vi "HEWH Mass Removed.vi"(8 "Error In":errorcluster, 11 "UEF Calculated Values Output in":T1 {"Data Indexes"."15 sec after Draw Index" format="%#.2f"; "Data Indexes"."15 sec after Draw Timestamp" format="%#.2f"; "Data Indexes"."Test Start Timestamp" format="%.2f"; "Data Indexes"."Test End Timestamp" format="%.2f"; "Data Indexes"."T0 Timestamp" format="%.2f"; "Data Indexes"."Tsf Timestamp" format="%.2f"; "Data Indexes"."Tsu0 Timestamp" format="%.2f"; "Data Indexes"."Tmax1 Timestamp" format="%.2f"; "Data Indexes"."Draw Index Timestamp" format="%#.2f"; "Data Indexes"."Non-Draw Timestamp" format="%#.2f"; "Data Indexes"."Heating Timestamp" format="%#.2f"; "Data Indexes"."Start Energy (BTU-Gas)" format="%.6f"; "Data Indexes"."Start Watt Hours" format="%.6f"; "Static Data"."V - Volume of Wh (True)" format="%.5f"; "Static Data"."T-Ambinet Nominal (°F)" format="%.5f"; "Static Data"."T-Inlet Setpoint (°F)" format="%.5f"; "Static Data"."T-Wh Setpoint (°F)" format="%.5f"; "Sampled Data"."Qe (Wh)" format="%.5f"; "Sampled Data"."Tau stby2 (hr)" format="%.5f"; "Sampled Data"."Tastby2 (°F)" format="%.5f"; "Sampled Data"."Qf (BTU)" format="%.5f"; "Sampled Data"."Qe (BTU)" format="%.5f"; "Sampled Data"."Tmax1 (°F)" format="%.5f"; "Sampled Data"."T0 (°F)" format="%.5f"; "Sampled Data"."Qr (BTU)" format="%.5f"; "Sampled Data"."T 24(°F)" format="%.5f"; "Sampled Data"."T astby(°F)" format="%.5f"; "Sampled Data"."T tstby(°F)" format="%.5f"; "Sampled Data"."T su0(°F)" format="%.5f"; "Sampled Data"."T suf(°F)" format="%.5f"; "Sampled Data"."Tau stby_1 (hr)" format="%.5f"; "Sampled Data"."Qsuf (BTU)" format="%.5f"; "Sampled Data"."Qsu0 (BTU)" format="%.5f"; "Calculated Values"."Draw Bonus Volume (gal)" format="%.6f"; "Calculated Values"."Adjustment Factor" format="%.6f"; "Calculated Values"."T*avg_del(n-1)" format="%.6f"; "Calculated Values"."T*min(n-1)" format="%.6f"; "Calculated Values"."T*avg_del(n)" format="%.6f"; "Calculated Values"."Vn" format="%.6f"; "Calculated Values"."Qdm (BTU)" format="%.6f"; "Calculated Values"."QHWD (BTU)" format="%.6f"; "Calculated Values"."QHW (BTU)" format="%.6f"; "Calculated Values"."UEF" format="%.6f"; "Calculated Values"."QHW67 (BTU)" format="%.6f"; "Calculated Values"."Qda (BTU)" format="%.6f"; "Calculated Values"."Qd (BTU)" format="%.6f"; "Calculated Values"."Q (BTU)" format="%.6f"; "Calculated Values"."UA (BTU/(hr*F))" format="%.6f"; "Calculated Values"."Qhr (BTU/hr)" format="%.6f"; "Calculated Values"."Qstby (BTU)" format="%.6f"; "Calculated Values"."nu_r" format="%.6f"; "Calculated Values"."CpUEF (BTU/(lb*F))" format="%.6f"; "Calculated Values"."rho_nu (lb/gal)" format="%.6f"; "Calculated Values"."V1- Vol (Gal)" format="%.6f"; "Calculated Values"."M cluster mass removed (lb)" format="%.6f"; "Calculated Values"."Cp theoretical (BTU/(lbm °F))" format="%.6f"; "Calculated Values"."Tin1 - Mean Inlet 1st Cluster (°F)" format="%.6f"; "Calculated Values"."Tdel1-Mean Outlet 1st Cluster(°F)" format="%.6f"; "Calculated Values"."Cp 24 (BTU/(lb*F))" format="%.6f"; "Calculated Values"."Cp standby (BTU/(lb*F))" format="%.6f"; "Calculated Values"."Cp2 (BTU/(lb*F))" format="%.6f"; "Calculated Values"."Cp1 (BTU/(lb*F))" format="%.6f"; "Calculated Values"."rho 24 (lb/gal)" format="%.6f"; "Calculated Values"."rho standby (lb/gal)" format="%.6f"; "Calculated Values"."rho 2 (lb/gal)" format="%.6f"; "Calculated Values"."Density of cold water All (lbm/gal)" format="%#.3g"; "Calculated Values"."CpHW (BTU/(lbm °F))" format="%#.3g"; "Calculated Values"."Density of hot water All (lbm/gal)" format="%#.3g"; "Calculated Values"."Mass of water All (lbm)" format="%#.3f"}) -> (0 "Error Out":errorcluster, 3 "UEF Calculated Values Output out":T1={"Calculated Values"={"Draw Cluster - Actual (Gal)"=[], "Mass of water All (lbm)"=[], "Density of hot water All (lbm/gal)"=[], "CpHW (BTU/(lbm °F))"=[], "rho 2 (lb/gal)"=0.0, "rho standby (lb/gal)"=0.0, "rho 24 (lb/gal)"=0.0, "Cp1 (BTU/(lb*F))"=0.0, "Cp2 (BTU/(lb*F))"=0.0, "Cp standby (BTU/(lb*F))"=0.0, "Cp 24 (BTU/(lb*F))"=0.0, "nu_r"=0.0, "Qstby (BTU)"=0.0, "Qhr (BTU/hr)"=0.0, "UA (BTU/(hr*F))"=0.0, "Q (BTU)"=0.0, "Qd (BTU)"=0.0, "Qda (BTU)"=0.0, "QHW67 (BTU)"=0.0, "UEF"=0.0, "Tdel1-Mean Outlet 1st Cluster(°F)"=0.0, "Tin1 - Mean Inlet 1st Cluster (°F)"=0.0, "Cp theoretical (BTU/(lbm °F))"=0.0, "M cluster mass removed (lb)"=0.0, "V1- Vol (Gal)"=0.0, "Test Data -Start to End (Full Index)"=[], "rho_nu (lb/gal)"=0.0, "Density of cold water All (lbm/gal)"=[], "CpUEF (BTU/(lb*F))"=0.0, "QHW (BTU)"=0.0, "QHWD (BTU)"=0.0, "Qdm (BTU)"=0.0, "FHD-After 1 Hour (String)"=[], "Vn"=0.0, "T*avg_del(n)"=0.0, "Max Location"=0, "T*min(n-1)"=0.0, "T*avg_del(n-1)"=0.0, "Temp Greater than T*min(n-1)"=FALSE, "Adjustment Factor"=0.0, "Draw Bonus Volume (gal)"=0.0, "Flow Type - End Condition"=enum."ForcedDrawAfterHour"}, "Sampled Data"={"Cold Water Draw Amounts-(Gal)"=[], "T del_all - Outlet Temps (°F)"=[], "T in_all - Inlet Temps (°F)"=[], "Qsu0 (BTU)"=14385.3, "Qsuf (BTU)"=15959.6, "Tau stby_1 (hr)"=8.4, "T suf(°F)"=125.0, "T su0(°F)"=126.1, "T tstby(°F)"=124.2, "T astby(°F)"=68.8, "T 24(°F)"=123.2, "Qr (BTU)"=7657.9, "T0 (°F)"=124.7, "Tmax1 (°F)"=124.8, "Qe (BTU)"=32770.2, "Qf (BTU)"=0.0, "Tastby2 (°F)"=68.9, "RTD Out Full Data\nSet (Each Draw)"=[], "RTD IN Full Data\nSet (Each Draw)"=[], "Tau stby2 (hr)"=23.406, "Hot Water Draw Amounts-(Gal)"=[], "Cold Flow Rate (GPM)"=[], "Hot Flow Rate (GPM)"=[], "Softw Elapsed Time\n Full Data Set (Each Draw)"=[], "Cold Gal Total Full\nData Set (Each Draw)"=[], "Total Hot Draw Amount (Gal) "=0.0, "Total Cold Draw Amount (Gal)"=0.0, "Qe (Wh)"=0.0, "Hot Gal Total Full\nData Set (Each Draw)"=[]}, "Static Data"={"T-Wh Setpoint (°F)"=125.0, "T-Inlet Setpoint (°F)"=58.0, "T-Ambinet Nominal (°F)"=67.5, "V - Volume of Wh (True)"=46.0}, "Data Indexes"={"Test Start-Full Index (Found)"=0, "Header Length"=0, "Draw Index (Found)"=[], "Nr"=0, "Start Watt Hours"=0.0, "Tsu0 Index (Found)"=0, "Tsf Index (Found)"=0, "Start Energy (BTU-Gas)"=0.0, "Draws in Cluster"=0, "T0 Index-Full Index (Found)"=0, "Non-Draw Index (Found)"=[], "Tmax1 Index (Found)"=0, "Test End-Full Index (Found)"=0, "Heating Index (Found)"=[], "Heating Timestamp"=[], "Non-Draw Timestamp"=[], "Draw Index Timestamp"=[], "Tmax1 Timestamp"=0.0, "Tsu0 Timestamp"=0.0, "Tsf Timestamp"=0.0, "T0 Timestamp"=0.0, "Test End Timestamp"=0.0, "Test Start Timestamp"=0.0, "15 sec after Draw Timestamp"=[], "15 sec after Draw Index"=[], "Tmax1 Occurred During a Draw"=FALSE, "FHD Total Time (Sec)"=0.0, "Draw Pattern"=enum."Very Small Usage", "Standby Valid"=FALSE}, "Raw Data"={"Elapsed Time Index (DBL)"=0, "Software Elapsed Time Index (DBL)"=0, "TC Tree Avg Index (DBL)"=0, "Watt Hours -Wh Index (DBL)"=0, "Energy BTU Index (DBL)"=0, "Totalized Flow Index (DBL)"=0, "Flow Rate Index (DBL)"=0, "Program Status Index (Str)"=0, "RTDin Index (DBL)"=0, "RTDout Index (DBL)"=0, "RTDamb Index (DBL)"=0, "Test Data-Start to End DBL"=[], "Data Type"=enum."GEA Inlet Side Meter", "Heat Source Index (DBL)"=0, "Hot Water Rate GPM (DBL)"=0, "Hot Water Total - GAL (DBL)"=0, "FHD-After 1 hour"=[], "Humidity -% RH (DBL)"=0, "Voltage - V (DBL)"=0, "Draw Count (DBL)"=0, "Elapsed Time Index (Str)"=0, "Software Elapsed Time Index (Str)"=0, "Frequency-Hz (Str)"=0, "RTDin Index (Str)"=0, "RTDout Index (Str)"=0, "RTDamb Index (Str)"=0, "UE (Str)"=0, "LE (Str)"=0, "Compressor (Str)"=0, "Flow Rate Index (Str)"=0, "Hot Water Total - GAL (Str)"=0}, "Tolerance Check (T)=Pass"={"Flow Rate"=FALSE, "Totalized Flow"=FALSE, "Ambient Temp (Full Range)"=FALSE, "Ambient Humidity (Full Range)"=FALSE, "Inlet Temp"=FALSE, "Outlet Temp"=FALSE, "Valid Test"=FALSE, "Individual Totalized Flow"=FALSE, "Data Sheet Check"="", "Inlet Temperature"=[], "Tinlet Max"=[], "Tinlet Min"=[], "Flow Rate Max (Tol)"=[], "Flow Rate Min (Tol)"=[], "Amb Temp Max"=0.0, "Amb Temp Min"=0.0, "Toutlet Max - Draw 1"=0.0, "Humidity Upper Tolerance (%)"=0.0, "Total Volume Tolerance (Gal)"=0.0, "Humidity Lower Tolerance (%)"=0.0, "Flow Rate Max\nPer Draw"=[], "Flow Rate Min\nPer Draw"=[], "Ambient Humidity (Runtime)"=FALSE, "Humidity Avg (Runtime)"=0.0, "Ambient Temp (On-Time AVG)"=FALSE, "Ambient Temp (Off-Time AVG)"=FALSE, "Amb Temp OFF Avg"=0.0, "Amb Temp ON Avg"=0.0, "Voltage (Heating)"=FALSE, "Voltage (Min)"=0.0, "Voltage (Max)"=0.0, "Toutlet Max"=[], "Toutlet Min"=[]}, "Test Information"={"TR Number"="", "Lab ID"="", "Notes/Config"="", "Model Number"="", "Serial Number"="", "Lab Technician"="", "Engineer"="", "Type of Fuel"="", "Samp Received Date"="", "Samp Test Date"="", "Report Date"="", "Rate Input (kW or BTU/hr)"="", "Measured Input (kW or BTU/hr)"="", "Filename"="", "Calibration Information"=[], "Calculator Version"="", "Minimum UEF Per CFR"=0.0, "UEF Report Information"=[], "FHR Report Information"=[], "FHR Front Panel Display"=[], "UEF Front Panel Display"=[], "Draw Outlet Temp Viewer"=[]}} {"Data Indexes"."15 sec after Draw Index" format="%#.2f"; "Data Indexes"."15 sec after Draw Timestamp" format="%#.2f"; "Data Indexes"."Test Start Timestamp" format="%.2f"; "Data Indexes"."Test End Timestamp" format="%.2f"; "Data Indexes"."T0 Timestamp" format="%.2f"; "Data Indexes"."Tsf Timestamp" format="%.2f"; "Data Indexes"."Tsu0 Timestamp" format="%.2f"; "Data Indexes"."Tmax1 Timestamp" format="%.2f"; "Data Indexes"."Draw Index Timestamp" format="%#.2f"; "Data Indexes"."Non-Draw Timestamp" format="%#.2f"; "Data Indexes"."Heating Timestamp" format="%#.2f"; "Data Indexes"."Start Energy (BTU-Gas)" format="%.6f"; "Data Indexes"."Start Watt Hours" format="%.6f"; "Static Data"."V - Volume of Wh (True)" format="%.5f"; "Static Data"."T-Ambinet Nominal (°F)" format="%.5f"; "Static Data"."T-Inlet Setpoint (°F)" format="%.5f"; "Static Data"."T-Wh Setpoint (°F)" format="%.5f"; "Sampled Data"."Qe (Wh)" format="%.5f"; "Sampled Data"."Tau stby2 (hr)" format="%.5f"; "Sampled Data"."Tastby2 (°F)" format="%.5f"; "Sampled Data"."Qf (BTU)" format="%.5f"; "Sampled Data"."Qe (BTU)" format="%.5f"; "Sampled Data"."Tmax1 (°F)" format="%.5f"; "Sampled Data"."T0 (°F)" format="%.5f"; "Sampled Data"."Qr (BTU)" format="%.5f"; "Sampled Data"."T 24(°F)" format="%.5f"; "Sampled Data"."T astby(°F)" format="%.5f"; "Sampled Data"."T tstby(°F)" format="%.5f"; "Sampled Data"."T su0(°F)" format="%.5f"; "Sampled Data"."T suf(°F)" format="%.5f"; "Sampled Data"."Tau stby_1 (hr)" format="%.5f"; "Sampled Data"."Qsuf (BTU)" format="%.5f"; "Sampled Data"."Qsu0 (BTU)" format="%.5f"; "Calculated Values"."Draw Bonus Volume (gal)" format="%.6f"; "Calculated Values"."Adjustment Factor" format="%.6f"; "Calculated Values"."T*avg_del(n-1)" format="%.6f"; "Calculated Values"."T*min(n-1)" format="%.6f"; "Calculated Values"."T*avg_del(n)" format="%.6f"; "Calculated Values"."Vn" format="%.6f"; "Calculated Values"."Qdm (BTU)" format="%.6f"; "Calculated Values"."QHWD (BTU)" format="%.6f"; "Calculated Values"."QHW (BTU)" format="%.6f"; "Calculated Values"."UEF" format="%.6f"; "Calculated Values"."QHW67 (BTU)" format="%.6f"; "Calculated Values"."Qda (BTU)" format="%.6f"; "Calculated Values"."Qd (BTU)" format="%.6f"; "Calculated Values"."Q (BTU)" format="%.6f"; "Calculated Values"."UA (BTU/(hr*F))" format="%.6f"; "Calculated Values"."Qhr (BTU/hr)" format="%.6f"; "Calculated Values"."Qstby (BTU)" format="%.6f"; "Calculated Values"."nu_r" format="%.6f"; "Calculated Values"."CpUEF (BTU/(lb*F))" format="%.6f"; "Calculated Values"."rho_nu (lb/gal)" format="%.6f"; "Calculated Values"."V1- Vol (Gal)" format="%.6f"; "Calculated Values"."M cluster mass removed (lb)" format="%.6f"; "Calculated Values"."Cp theoretical (BTU/(lbm °F))" format="%.6f"; "Calculated Values"."Tin1 - Mean Inlet 1st Cluster (°F)" format="%.6f"; "Calculated Values"."Tdel1-Mean Outlet 1st Cluster(°F)" format="%.6f"; "Calculated Values"."Cp 24 (BTU/(lb*F))" format="%.6f"; "Calculated Values"."Cp standby (BTU/(lb*F))" format="%.6f"; "Calculated Values"."Cp2 (BTU/(lb*F))" format="%.6f"; "Calculated Values"."Cp1 (BTU/(lb*F))" format="%.6f"; "Calculated Values"."rho 24 (lb/gal)" format="%.6f"; "Calculated Values"."rho standby (lb/gal)" format="%.6f"; "Calculated Values"."rho 2 (lb/gal)" format="%.6f"; "Calculated Values"."Density of cold water All (lbm/gal)" format="%#.3g"; "Calculated Values"."CpHW (BTU/(lbm °F))" format="%#.3g"; "Calculated Values"."Density of hot water All (lbm/gal)" format="%#.3g"; "Calculated Values"."Mass of water All (lbm)" format="%#.3f"})   [LabVIEW 2023]
uses:
  Type Definitions/UEF Constants.ctl
  Type Definitions/HEWH Draw Stats.ctl
  Type Definitions/HEWH FHR Draw Type.ctl
  Type Definitions/FHR Bins.ctl
  Type Definitions/HEWH Meter Type.ctl
panel:
  # "FHR"
  # "FHR"
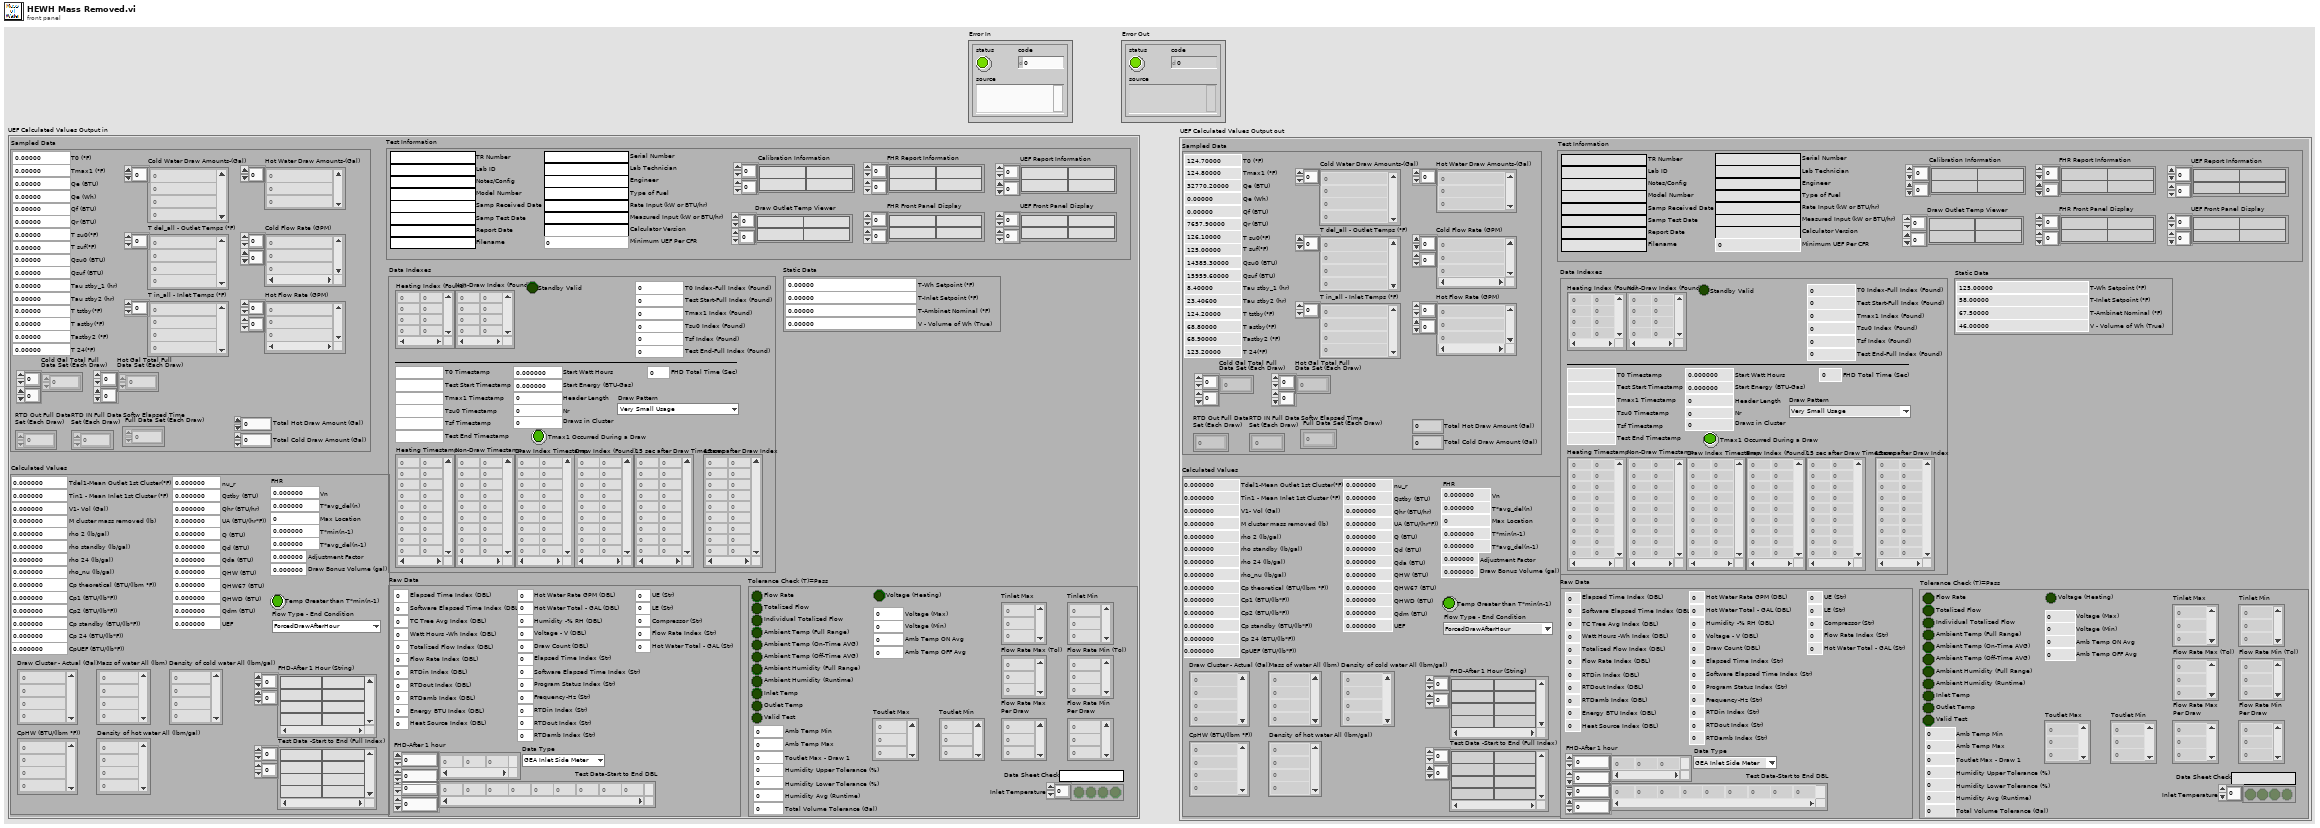
[diagram p1: front panel]
types:
  T1 = typedef "UEF Constants.ctl" = cluster{"Calculated Values":T2, "Sampled Data":cluster{"Cold Water Draw Amounts-(Gal)":dbl[], "T del_all - Outlet Temps (°F)":dbl[], "T in_all - Inlet Temps (°F)":dbl[], "Qsu0 (BTU)":dbl, "Qsuf (BTU)":dbl, "Tau stby_1 (hr)":dbl, "T suf(°F)":dbl, "T su0(°F)":dbl, "T tstby(°F)":dbl, "T astby(°F)":dbl, "T 24(°F)":dbl, "Qr (BTU)":dbl, "T0 (°F)":dbl, "Tmax1 (°F)":dbl, "Qe (BTU)":dbl, "Qf (BTU)":dbl, "Tastby2 (°F)":dbl, "RTD Out Full Data\nSet (Each Draw)":dbl[][], "RTD IN Full Data\nSet (Each Draw)":dbl[][], "Tau stby2 (hr)":dbl, "Hot Water Draw Amounts-(Gal)":dbl[], "Cold Flow Rate (GPM)":dbl[][], "Hot Flow Rate (GPM)":dbl[][], "Softw Elapsed Time\n Full Data Set (Each Draw)":dbl[][], "Cold Gal Total Full\nData Set (Each Draw)":dbl[][], "Total Hot Draw Amount (Gal) ":dbl, "Total Cold Draw Amount (Gal)":dbl, "Qe (Wh)":dbl, "Hot Gal Total Full\nData Set (Each Draw)":dbl[][]}, "Static Data":cluster{"T-Wh Setpoint (°F)":dbl, "T-Inlet Setpoint (°F)":dbl, "T-Ambinet Nominal (°F)":dbl, "V - Volume of Wh (True)":dbl}, "Data Indexes":cluster{"Test Start-Full Index (Found)":i32, "Header Length":i32, "Draw Index (Found)":i32[][], "Nr":i32, "Start Watt Hours":dbl, "Tsu0 Index (Found)":i32, "Tsf Index (Found)":i32, "Start Energy (BTU-Gas)":dbl, "Draws in Cluster":i32, "T0 Index-Full Index (Found)":i32, "Non-Draw Index (Found)":i32[][], "Tmax1 Index (Found)":i32, "Test End-Full Index (Found)":i32, "Heating Index (Found)":i32[][], "Heating Timestamp":dbl[][], "Non-Draw Timestamp":dbl[][], "Draw Index Timestamp":dbl[][], "Tmax1 Timestamp":dbl, "Tsu0 Timestamp":dbl, "Tsf Timestamp":dbl, "T0 Timestamp":dbl, "Test End Timestamp":dbl, "Test Start Timestamp":dbl, "15 sec after Draw Timestamp":dbl[][], "15 sec after Draw Index":dbl[][], "Tmax1 Occurred During a Draw":bool, "FHD Total Time (Sec)":dbl, "Draw Pattern":T4, "Standby Valid":bool}, "Raw Data":cluster{"Elapsed Time Index (DBL)":i32, "Software Elapsed Time Index (DBL)":i32, "TC Tree Avg Index (DBL)":i32, "Watt Hours -Wh Index (DBL)":i32, "Energy BTU Index (DBL)":i32, "Totalized Flow Index (DBL)":i32, "Flow Rate Index (DBL)":i32, "Program Status Index (Str)":i32, "RTDin Index (DBL)":i32, "RTDout Index (DBL)":i32, "RTDamb Index (DBL)":i32, "Test Data-Start to End DBL":dbl[][], "Data Type":T5, "Heat Source Index (DBL)":i32, "Hot Water Rate GPM (DBL)":i32, "Hot Water Total - GAL (DBL)":i32, "FHD-After 1 hour":dbl[][], "Humidity -% RH (DBL)":i32, "Voltage - V (DBL)":i32, "Draw Count (DBL)":i32, "Elapsed Time Index (Str)":i32, "Software Elapsed Time Index (Str)":i32, "Frequency-Hz (Str)":i32, "RTDin Index (Str)":i32, "RTDout Index (Str)":i32, "RTDamb Index (Str)":i32, "UE (Str)":i32, "LE (Str)":i32, "Compressor (Str)":i32, "Flow Rate Index (Str)":i32, "Hot Water Total - GAL (Str)":i32}, "Tolerance Check (T)=Pass":cluster{"Flow Rate":bool, "Totalized Flow":bool, "Ambient Temp (Full Range)":bool, "Ambient Humidity (Full Range)":bool, "Inlet Temp":bool, "Outlet Temp":bool, "Valid Test":bool, "Individual Totalized Flow":bool, "Data Sheet Check":string, "Inlet Temperature":bool[], "Tinlet Max":dbl[], "Tinlet Min":dbl[], "Flow Rate Max (Tol)":dbl[], "Flow Rate Min (Tol)":dbl[], "Amb Temp Max":dbl, "Amb Temp Min":dbl, "Toutlet Max - Draw 1":dbl, "Humidity Upper Tolerance (%)":dbl, "Total Volume Tolerance (Gal)":dbl, "Humidity Lower Tolerance (%)":dbl, "Flow Rate Max\nPer Draw":dbl[], "Flow Rate Min\nPer Draw":dbl[], "Ambient Humidity (Runtime)":bool, "Humidity Avg (Runtime)":dbl, "Ambient Temp (On-Time AVG)":bool, "Ambient Temp (Off-Time AVG)":bool, "Amb Temp OFF Avg":dbl, "Amb Temp ON Avg":dbl, "Voltage (Heating)":bool, "Voltage (Min)":dbl, "Voltage (Max)":dbl, "Toutlet Max":dbl[], "Toutlet Min":dbl[]}, "Test Information":cluster{"TR Number":string, "Lab ID":string, "Notes/Config":string, "Model Number":string, "Serial Number":string, "Lab Technician":string, "Engineer":string, "Type of Fuel":string, "Samp Received Date":string, "Samp Test Date":string, "Report Date":string, "Rate Input (kW or BTU/hr)":string, "Measured Input (kW or BTU/hr)":string, "Filename":string, "Calibration Information":string[][], "Calculator Version":string, "Minimum UEF Per CFR":dbl, "UEF Report Information":string[][], "FHR Report Information":string[][], "FHR Front Panel Display":string[][], "UEF Front Panel Display":string[][], "Draw Outlet Temp Viewer":string[][]}}
  T2 = typedef "HEWH Draw Stats.ctl" = cluster{"Draw Cluster - Actual (Gal)":dbl[], "Mass of water All (lbm)":dbl[], "Density of hot water All (lbm/gal)":dbl[], "CpHW (BTU/(lbm °F))":dbl[], "rho 2 (lb/gal)":dbl, "rho standby (lb/gal)":dbl, "rho 24 (lb/gal)":dbl, "Cp1 (BTU/(lb*F))":dbl, "Cp2 (BTU/(lb*F))":dbl, "Cp standby (BTU/(lb*F))":dbl, "Cp 24 (BTU/(lb*F))":dbl, "nu_r":dbl, "Qstby (BTU)":dbl, "Qhr (BTU/hr)":dbl, "UA (BTU/(hr*F))":dbl, "Q (BTU)":dbl, "Qd (BTU)":dbl, "Qda (BTU)":dbl, "QHW67 (BTU)":dbl, "UEF":dbl, "Tdel1-Mean Outlet 1st Cluster(°F)":dbl, "Tin1 - Mean Inlet 1st Cluster (°F)":dbl, "Cp theoretical (BTU/(lbm °F))":dbl, "M cluster mass removed (lb)":dbl, "V1- Vol (Gal)":dbl, "Test Data -Start to End (Full Index)":string[][], "rho_nu (lb/gal)":dbl, "Density of cold water All (lbm/gal)":dbl[], "CpUEF (BTU/(lb*F))":dbl, "QHW (BTU)":dbl, "QHWD (BTU)":dbl, "Qdm (BTU)":dbl, "FHD-After 1 Hour (String)":string[][], "Vn":dbl, "T*avg_del(n)":dbl, "Max Location":i32, "T*min(n-1)":dbl, "T*avg_del(n-1)":dbl, "Temp Greater than T*min(n-1)":bool, "Adjustment Factor":dbl, "Draw Bonus Volume (gal)":dbl, "Flow Type - End Condition":T3}
  T3 = typedef "HEWH FHR Draw Type.ctl" = enum16{"ForcedDrawAfterHour", "HeatingCutoffBeforeHour"}
  T4 = typedef "FHR Bins.ctl" = enum16{"Very Small Usage", "Low Usage", "Medium Usage", "High Usage", "Undefined"}
  T5 = typedef "HEWH Meter Type.ctl" = enum16{"GEA Inlet Side Meter", "GEA Outlet Side Meter", "CSA Inlet Side Meter"}
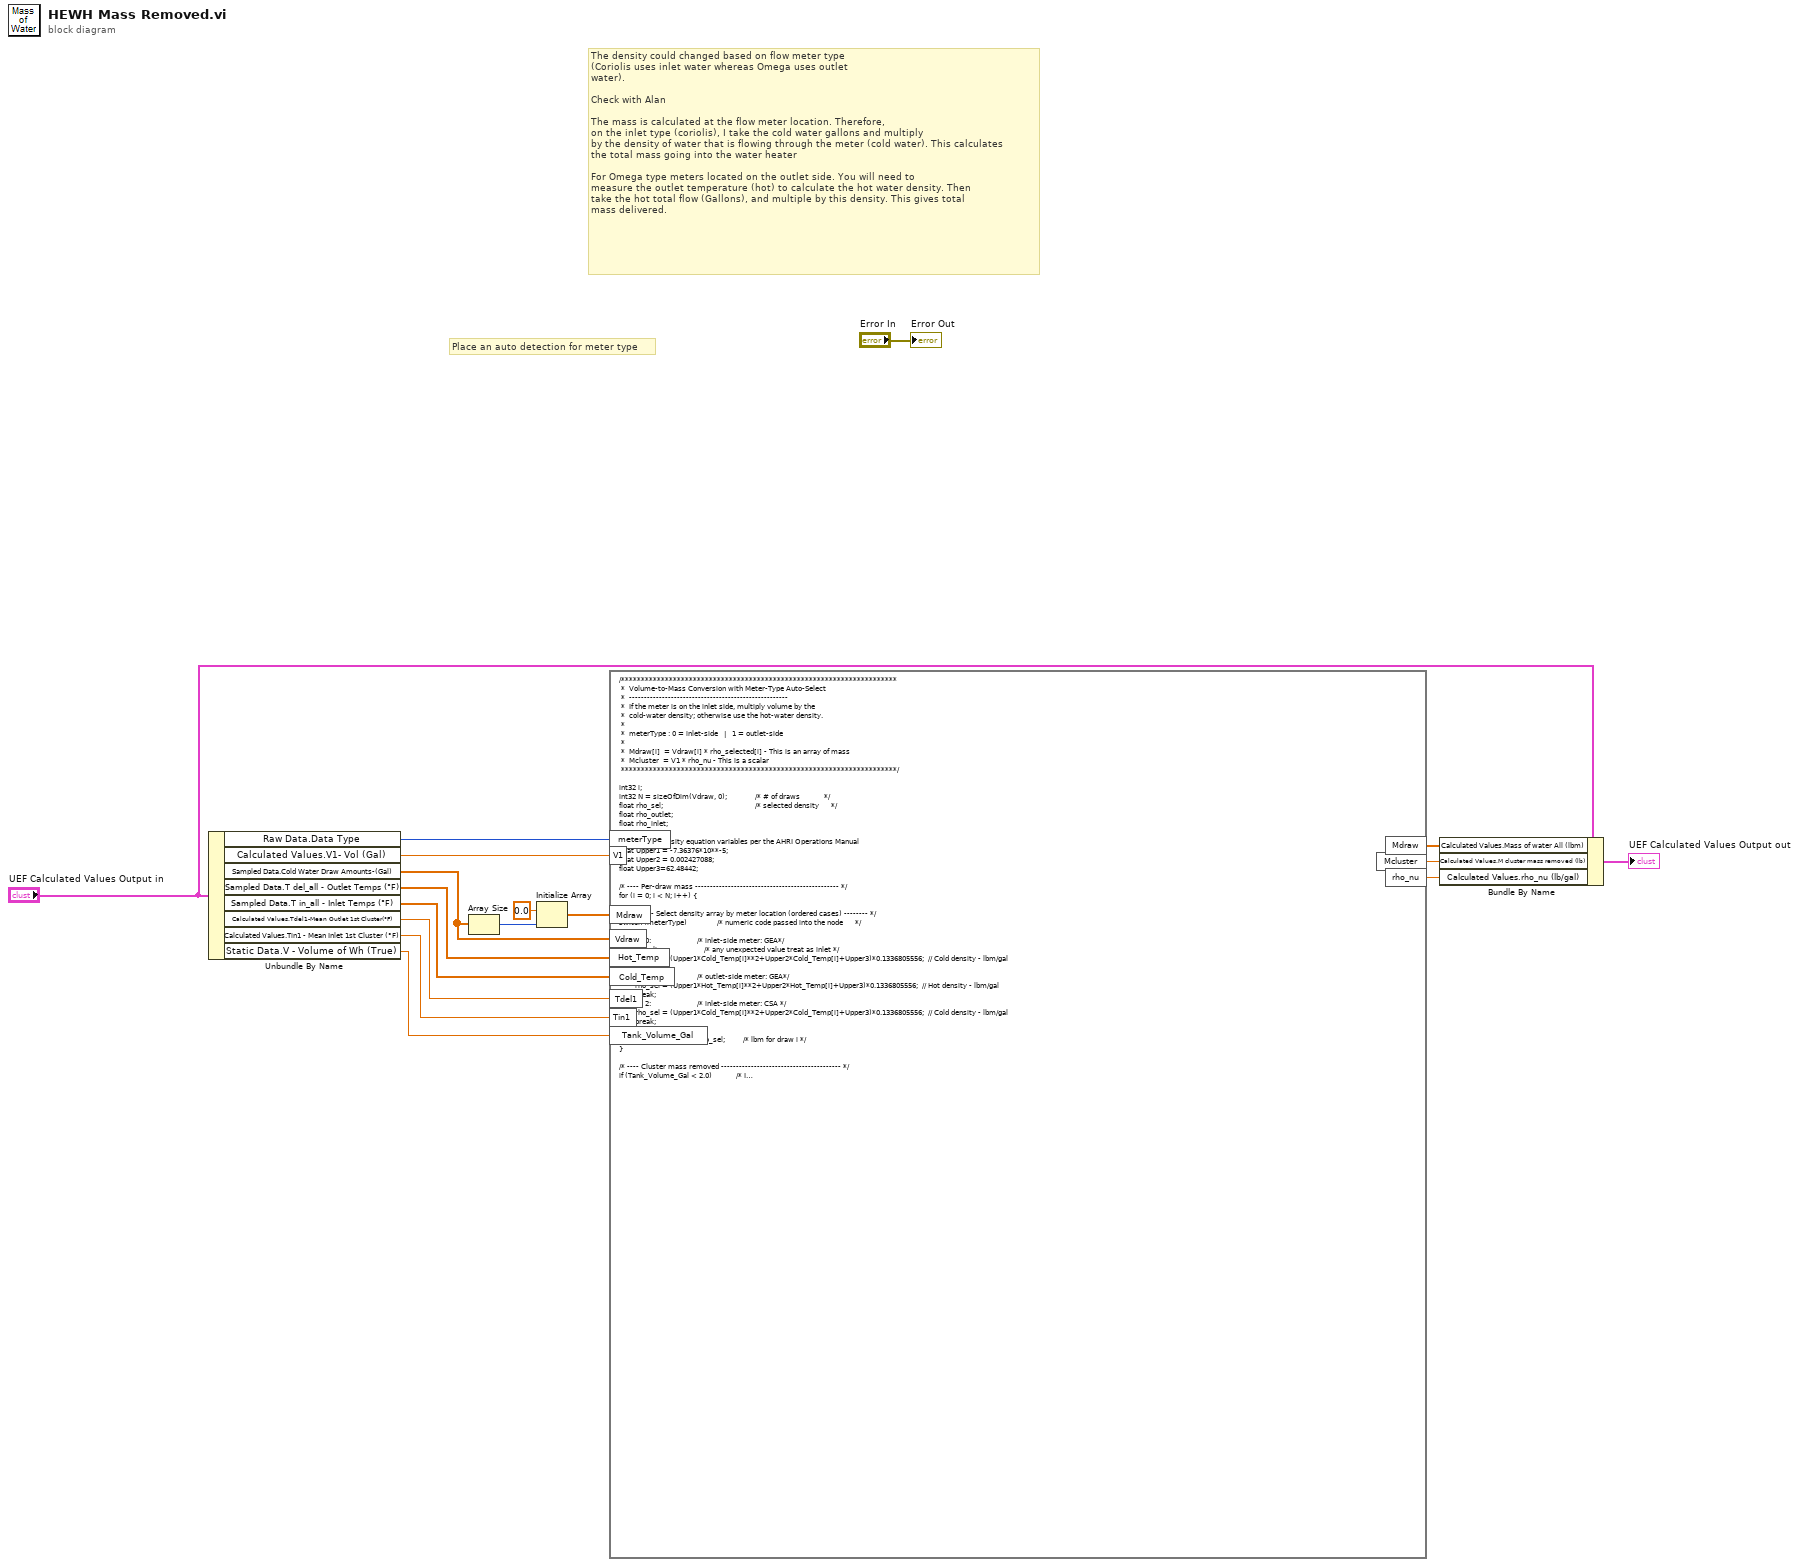
[diagram p0: block diagram]
diagram:
  # "Place an auto detection for meter type"
  # "The density could changed based on flow meter type\n(Coriolis uses inlet water whereas Omega uses outlet \nwater).\n\nCheck with Alan\n\nThe mass is calculated at the flow meter location. Therefore, \non the inlet type (coriolis), I take the cold water gallons and multiply\nby the density of water that is flowing through the meter (cold water). This calculates\nthe total mass going into the water heater\n\nFor Omega type meters located on the outlet side. You will need to \nmeasure the outlet temperature (hot) to calculate the hot water density. Then \ntake the hot total flow (Gallons), and multiple by this density. This gives total\nmass delivered."
  n1 = Unbundle By Name("UEF Calculated Values Output in") -> ("Raw Data.Data Type"=w14:T5, "Calculated Values.V1- Vol (Gal)"=w13:dbl, "Sampled Data.Cold Water Draw Amounts-(Gal)"=w5:dbl[], "Sampled Data.T del_all - Outlet Temps (°F)"=w7:dbl[], "Sampled Data.T in_all - Inlet Temps (°F)"=w6:dbl[], "Calculated Values.Tdel1-Mean Outlet 1st Cluster(°F)"=w4:dbl, "Calculated Values.Tin1 - Mean Inlet 1st Cluster (°F)"=w3:dbl, "Static Data.V - Volume of Wh (True)"=w2:dbl)
  n2 = Array Size(array=w5) -> (size(s)=w12:i32)
  n3 = Initialize Array(0.0 ("element"), w12) -> (w10:dbl[])
  n4 = formula code="/*********************************************************************\n *  Volume-to-Mass Conversion with Meter-Type Auto-Select\n *  -----------------------------------------------------\n *  If the meter is on the inlet side, multiply volume by the\n *  cold-water density; otherwise use the hot-water density.\n *\n *  meterType : 0 = inlet-side   |   1 = outlet-side\n *\n *  Mdraw[i]  = Vdraw[i] * rho_selected[i] - This is an array of mass\n *  Mcluster  = V1 * rho_nu - This is a scalar\n *********************************************************************/\n\nint32 i;\nint32 N = sizeOfDim(Vdraw, 0);              /* # of draws            */\nfloat rho_sel;                                              /* selected density      */\nfloat rho_outlet;\nfloat rho_inlet;\n\n//Define the density equation variables per the AHRI Operations Manual\nfloat Upper1 = -7.36376*10**-5;\nfloat Upper2 = 0.002427088;\nfloat Upper3=62.48442;\n\n/* ---- Per-draw mass ------------------------------------------------ */\nfor (i = 0; i < N; i++) {\n\n/* --------- Select density array by meter location (ordered cases) -------- */\nswitch (meterType)               /* numeric code passed into the node      */\n{\n    case 0:                       /* inlet-side meter: GEA*/\n        default:                      /* any unexpected value treat as inlet */\n        rho_sel = (Upper1*Cold_Temp[i]**2+Upper2*Cold_Temp[i]+Upper3)*0.1336805556;  // Cold density - lbm/gal\n        break;\n    case 1:                       /* outlet-side meter: GEA*/\n        rho_sel = (Upper1*Hot_Temp[i]**2+Upper2*Hot_Temp[i]+Upper3)*0.1336805556;  // Hot density - lbm/gal\n        break;\n    case 2:                       /* inlet-side meter: CSA */\n        rho_sel = (Upper1*Cold_Temp[i]**2+Upper2*Cold_Temp[i]+Upper3)*0.1336805556;  // Cold density - lbm/gal\n        break;\n}\nMdraw[i] = Vdraw[i] * rho_sel;         /* lbm for draw i */\n}\n\n/* ---- Cluster mass removed ---------------------------------------- */\nif (Tank_Volume_Gal < 2.0)            /* Instantaneous / very-small */\n{\n   rho_nu = (Upper1*Tdel1**2+Upper2*Tdel1+Upper3)*0.1336805556;  // density - lbm/gal\n   Mcluster = V1 * rho_nu;                 /* lb  (= gal × lb/gal)     */\n}\nelse                                                     /* Storage Water Heater*/\n{\n   rho_outlet = (Upper1*Tdel1**2+Upper2*Tdel1+Upper3)*0.1336805556;  // density - lbm/gal\n   rho_inlet = (Upper1*Tin1**2+Upper2*Tin1+Upper3)*0.1336805556;  // density - lbm/gal\n   rho_nu = (rho_outlet + rho_inlet)/2;\n\n   Mcluster = V1 * rho_nu;                 /* lb  (= gal × lb/gal)     */\n}"("meterType"=w14, "Vdraw"=w5, "V1"=w13, "Mdraw"=w10, "Hot_Temp"=w7, "Cold_Temp"=w6, "Tdel1"=w4, "Tin1"=w3, "Tank_Volume_Gal"=w2) -> ("Mcluster"=w8:dbl, "Mdraw"=w9:dbl[], "rho_nu"=w1:dbl)
  n5 = Bundle By Name(cluster="UEF Calculated Values Output in", "Calculated Values.Mass of water All (lbm)"=w9, "Calculated Values.M cluster mass removed (lb)"=w8, "Calculated Values.rho_nu (lb/gal)"=w1) -> (→"UEF Calculated Values Output out":T1)
  "Error Out" <- "Error In"
